vi "Lookup Frame.vi"(8 "error in (no error)":errorcluster, 10 "Frame":string, 11 "Ethernet in":refnum<class "ENET_BS120x.lvclass">) -> (0 "error out":errorcluster, 2 "XNET Frame":refnum<k21>, 3 "Ethernet out":refnum<class "ENET_BS120x.lvclass">)   [LabVIEW 2021, in "BS120x Driver.lvlib" / "ENET_BS120x.lvclass"]
uses:
  ENET_BS120x.lvclass
  ENET_BS120x.lvclass/ENET_BS120x.ctl
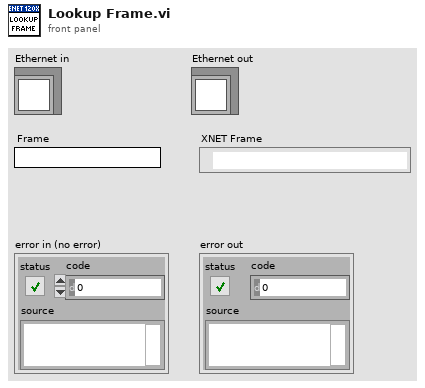
[diagram p1: front panel]
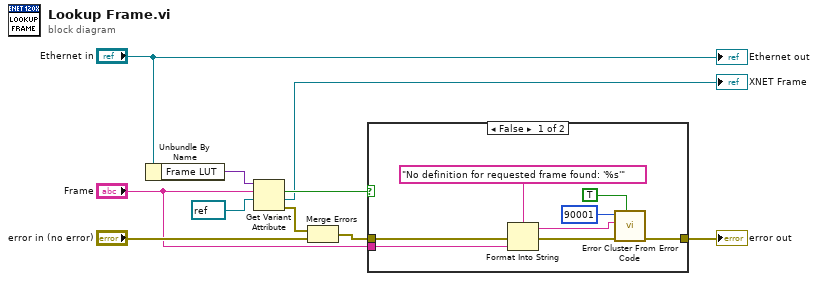
[diagram p0: block diagram]
diagram:
  n1 = Unbundle By Name("Ethernet in") -> ("Frame LUT"=w8:variant)
  n2 = Get Variant Attribute(Variant=w8, name="Frame", default value (empty Variant)=refnum<k21> refnum ("XNET Frame")) -> (found=w3:bool, value=→"XNET Frame":refnum<k21>, error out=w9:errorcluster)  [unwired: 1 in, 1 out]
  n3 = Merge Errors(w9, "error in (no error)") -> (w5:errorcluster)
  n4 = case shown="False" w3 {
    tunnel: w5 -> [w13 w19]
    tunnel: [w12 w19] -> w4
    tunnel: "Frame" -> [w11 _]
    frame False {
      n5 = Format Into String(format string="No definition for requested frame found: '%s'" ("source"), error in=w13, w11) -> (resulting string=w17:string, error out=w16:errorcluster)  [unwired: 1 in]
      n6 = call <vilib>:"Error Cluster From Error Code.vi"("show call chain? (False)"=TRUE, "error in (no error)"=w16, "error message (\"\")"=w17, "error code (0)"=90001) -> ("error out"=w12:errorcluster)  [unwired: 5 in]
    }
    frame True {
    }
  }
  "error out" <- w4
  "Ethernet out" <- "Ethernet in"
